vi "Close.vi"(0 "VISA resource name":refnum<visa-resource-name>, 11 "error in (no error)":errorcluster) -> (15 "error out":errorcluster)   [LabVIEW 2013, in "Fluke 5XXX Series Multicalibrators.lvlib"]
doc: "This VI closes the I/O interface with the instrument."
uses:
  Fluke 5XXX Series Multicalibrators.lvlib
  <vilib>/Instr/_visa.llb/VISA GPIB Control REN Mode.ctl
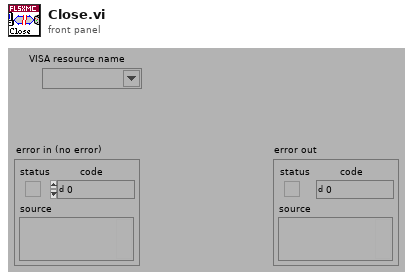
[diagram p1: front panel]
types:
  T1 = typedef "VISA GPIB Control REN Mode.ctl" = u16
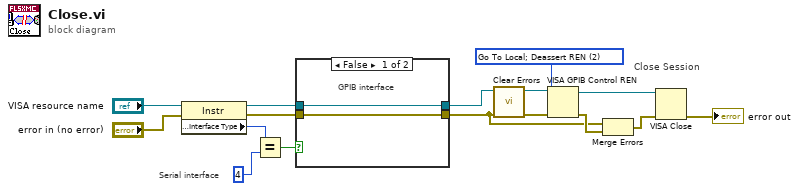
[diagram p0: block diagram]
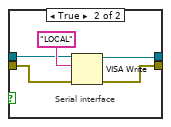
[diagram p2: hidden frame]
diagram:
  w5 = T1 2 items=["Deassert REN", "Assert REN", "Go To Local; Deassert REN ", "Assert REN; Address Device", "Local Lockout (Addressed Devices)", "Local Lockout (This Device)", "Go To Local"] ("Mode")
  # "Serial interface"
  # "Close Session"
  n1 = property class="Instr"(reference="VISA resource name", error in="error in (no error)") -> (reference out=w11:refnum<visa-resource-name>, error out=w12:errorcluster, "Interface Information:Interface Type"=w14:u16)
  n2 = Equal?(x=w14, y=u16 4) -> (x = y?=w13:bool)
  n3 = case shown="False" w13 {
    tunnel: w12 -> [w16 w20]
    tunnel: w11 -> [w17 w19]
    tunnel: [w16 w18] -> w3
    tunnel: [w17 w21] -> w6
    frame False {
      # "GPIB interface"
    }
    frame True {
      # "Serial interface"
      n4 = VISA Write(VISA resource name=w19, write buffer="LOCAL" ("ID Query"), error in (no error)=w20) -> (VISA resource name out=w21:refnum<visa-resource-name>, error out=w18:errorcluster)  [unwired: 1 out]
    }
  }
  n5 = call <vilib>:"Clear Errors.vi"("error in (no error)"=w3) -> ("error out"=w7:errorcluster)  [unwired: 6 in]
  n6 = VISA GPIB Control REN(8:w7, 10:w5, 11:w6) -> (0:w4:errorcluster, 3:w1:refnum<visa-resource-name>)
  n7 = Merge Errors(w3, w4) -> (w2:errorcluster)
  n8 = VISA Close(VISA resource name=w1, error in (no error)=w2) -> (error out=→"error out":errorcluster)
